vi "unregisterUserEvent.vi"(8 "error in (no error)":errorcluster, 11 "tcpServer in":refnum<class "TcpServer.lvclass">) -> (0 "error out":errorcluster, 3 "tcpServer out":refnum<class "TcpServer.lvclass">)   [LabVIEW 2018, in "TcpServer.lvclass"]
doc: "Unregister User Events."
uses:
  TcpServer.lvclass
  TcpServer.lvclass/TcpServer.ctl
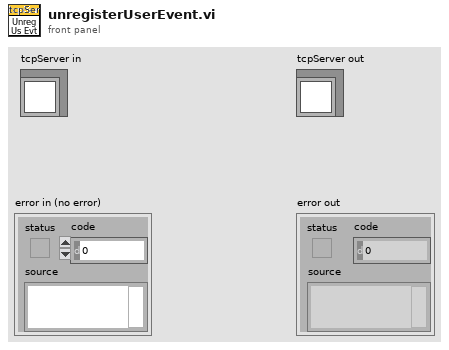
[diagram p1: front panel]
types:
  T1 = typedef "TcpServer.lvclass/userEventTypeDef.ctl" = cluster{"TcpServer":refnum<user-event>, "CmdRead":refnum<user-event>, "CmdWrite":refnum<user-event>, "MsgRead":refnum<user-event>, "MsgWrite":refnum<user-event>, "GenRead":refnum<user-event>, "GenWrite":refnum<user-event>}
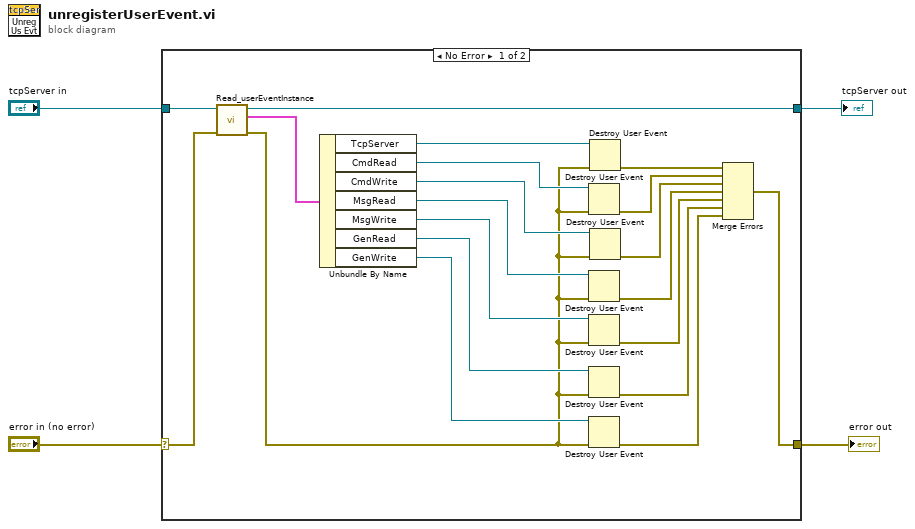
[diagram p0: block diagram]
diagram:
  n1 = case shown="No Error" "error in (no error)" {
    selector: "error in (no error)" -> [w22 w26]
    tunnel: [w18 w26] -> w3
    tunnel: [w23 w25] -> w1
    tunnel: "tcpServer in" -> [w24 w25]
    frame No Error {
      n2 = call "Read_userEventInstance.vi"("error in (no error)"=w22, "tcpServer in"=w24) -> ("error out"=w7:errorcluster, "UserEvents"=w20:T1, "tcpServer out"=w23:refnum<class "TcpServer.lvclass">)  [unwired: 7 in]
      n3 = Unbundle By Name(w20) -> ("TcpServer"=w19:refnum<user-event>, "CmdRead"=w16:refnum<user-event>, "CmdWrite"=w15:refnum<user-event>, "MsgRead"=w14:refnum<user-event>, "MsgWrite"=w12:refnum<user-event>, "GenRead"=w11:refnum<user-event>, "GenWrite"=w10:refnum<user-event>)
      n4 = Destroy User Event(user event=w16, error in=w7) -> (error out=w17:errorcluster)
      n5 = Destroy User Event(user event=w14, error in=w7) -> (error out=w9:errorcluster)
      n6 = Destroy User Event(user event=w12, error in=w7) -> (error out=w8:errorcluster)
      n7 = Destroy User Event(user event=w11, error in=w7) -> (error out=w6:errorcluster)
      n8 = Destroy User Event(user event=w10, error in=w7) -> (error out=w5:errorcluster)
      n9 = Destroy User Event(user event=w19, error in=w7) -> (error out=w21:errorcluster)
      n10 = Destroy User Event(user event=w15, error in=w7) -> (error out=w13:errorcluster)
      n11 = Merge Errors(w21, w17, w13, w9, w8, w6, w5) -> (w18:errorcluster)
    }
    frame Error {
    }
  }
  "error out" <- w3
  "tcpServer out" <- w1
